vi "Check and Override Channel Configuration.vi"(8 "error in (no error)":errorcluster, 10 "Custom Config Data in":u8[](array[numeric]) format="%.0x", 11 "CIF_NIChn_FIFO_DAQ in":refnum<class "CIF_NIChn_FIFO_DAQ.lvclass">) -> (0 "error out":errorcluster, 2 "Custom Config Data out":u8[](array[numeric]) format="%.0x", 3 "CIF_NIChn_FIFO_DAQ out":refnum<class "CIF_NIChn_FIFO_DAQ.lvclass">)   [LabVIEW 2021, in "CIF_NIChn_FIFO_DAQ.lvclass"]
uses:
  CIF_NIChn_FIFO_DAQ.lvclass
  <vilib>/CIF Foundation/CIF Utilities/DataTypes/Unflatten U64.vi
  <vilib>/CIF Foundation/CIF Utilities/DataTypes/Flatten U64.vi
  CIF_NIChn_FIFO_DAQ.lvclass/CIF_NIChn_FIFO_DAQ.ctl
  ChannelCommon/ChannelCommon.lvlib
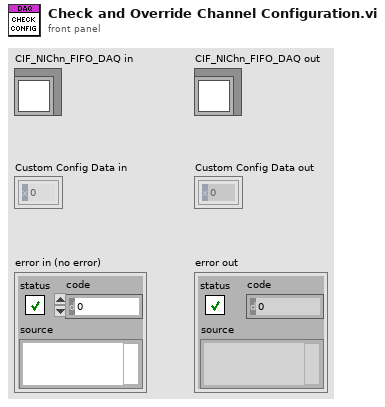
[diagram p1: front panel]
types:
  T1 = typedef "ChannelCommon.lvlib/FIFO Config.ctl" = cluster{"Max Bytes/Msg":u64, "Max Msg/FIFO":u64, "Flags":u64}
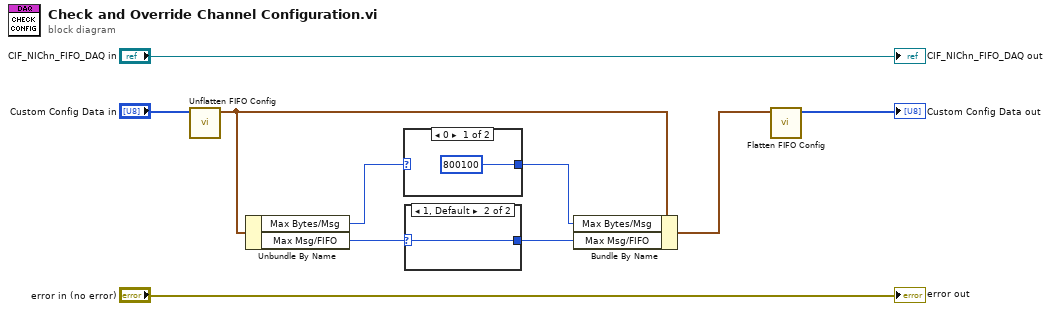
[diagram p0: block diagram]
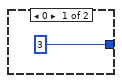
[diagram p3: hidden frame]
diagram:
  n1 = call "Unflatten FIFO Config.vi"("Flattened Data in"="Custom Config Data in") -> ("FIFO Config out"=w5:T1)  [unwired: 9 in, 1 out]
  n2 = Unbundle By Name(w5) -> ("Max Bytes/Msg"=w1:u64, "Max Msg/FIFO"=w4:u64)
  n3 = case shown="0" w1 {
    selector: w1 -> [_ w12]
    tunnel: [u64 800100 ("y") w12] -> w2
    frame 0 {
    }
    frame 1, Default {
    }
  }
  n4 = case shown="1, Default" w4 {
    selector: w4 -> [_ w14]
    tunnel: [u64 3 ("y") w14] -> w3
    frame 0 {
    }
    frame 1, Default {
    }
  }
  n5 = Bundle By Name(cluster=w5, "Max Bytes/Msg"=w2, "Max Msg/FIFO"=w3) -> (w6:T1)
  n6 = call "Flatten FIFO Config.vi"("FIFO Config in"=w6) -> ("Flattened FIFO Config"=→"Custom Config Data out":u8[])  [unwired: 10 in]
  "error out" <- "error in (no error)"
  "CIF_NIChn_FIFO_DAQ out" <- "CIF_NIChn_FIFO_DAQ in"
